vi "Initialize.vi"(7 "Serial Configuration":T1={"Baud Rate"=9600, "Parity"=0, "Data Bits"=8, "Stop Bits"=10, "Flow Control"=0} {"Flow Control" items=["None", "XON/XOFF", "RTS/CTS", "XON/XOFF & RTS/CTS", "DTR/DSR", "XON/XOFF & DTR/DSR"]; "Stop Bits" items=["1.0"=10, "1.5"=15, "2.0"=20]; "Data Bits" items=["7"=7, "8"=8]; "Parity" items=["None", "Odd", "Even", "Mark", "Space"]; "Baud Rate" items=["300"=300, "600"=600, "1200"=1200, "2400"=2400, "4800"=4800, "9600"=9600, "19200"=19200]}, 8 "error in (no error)":errorcluster, 9 "Reset (True)":bool=TRUE, 10 "ID Query (True)":bool=TRUE, 11 "VISA resource name":refnum<visa-resource-name>) -> (0 "error out":errorcluster, 3 "VISA resource name out":refnum<visa-resource-name>)   [LabVIEW 2014, in "Fluke 884X Series.lvlib"]
doc: "Establishes communication with the instrument and optionally performs an instrument identification query and/or an instrument reset. It also places the instrument in a default state needed for other instrument driver operations. Therefore, call this VI before calling other instrument driver VIs for this instrument. Generally, you need to call the <B>Initialize VI</B> only once at the beginning of an application."
uses:
  Fluke 884X Series.lvlib
panel:
  # "(c) 2007 National Instruments.  ALL RIGHTS RESERVED."
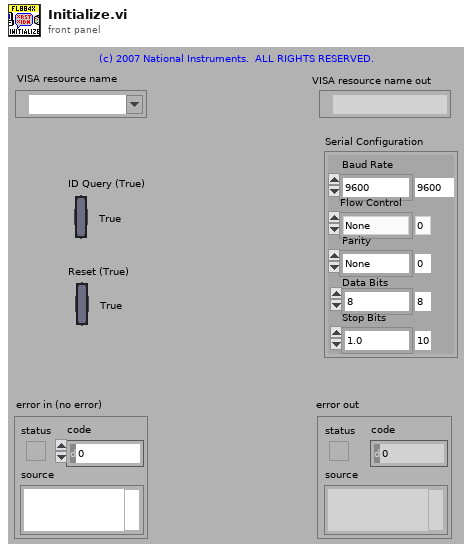
[diagram p1: front panel]
types:
  T1 = cluster{"Baud Rate":u32, "Parity":u16, "Data Bits":u16, "Stop Bits":u16, "Flow Control":u16}
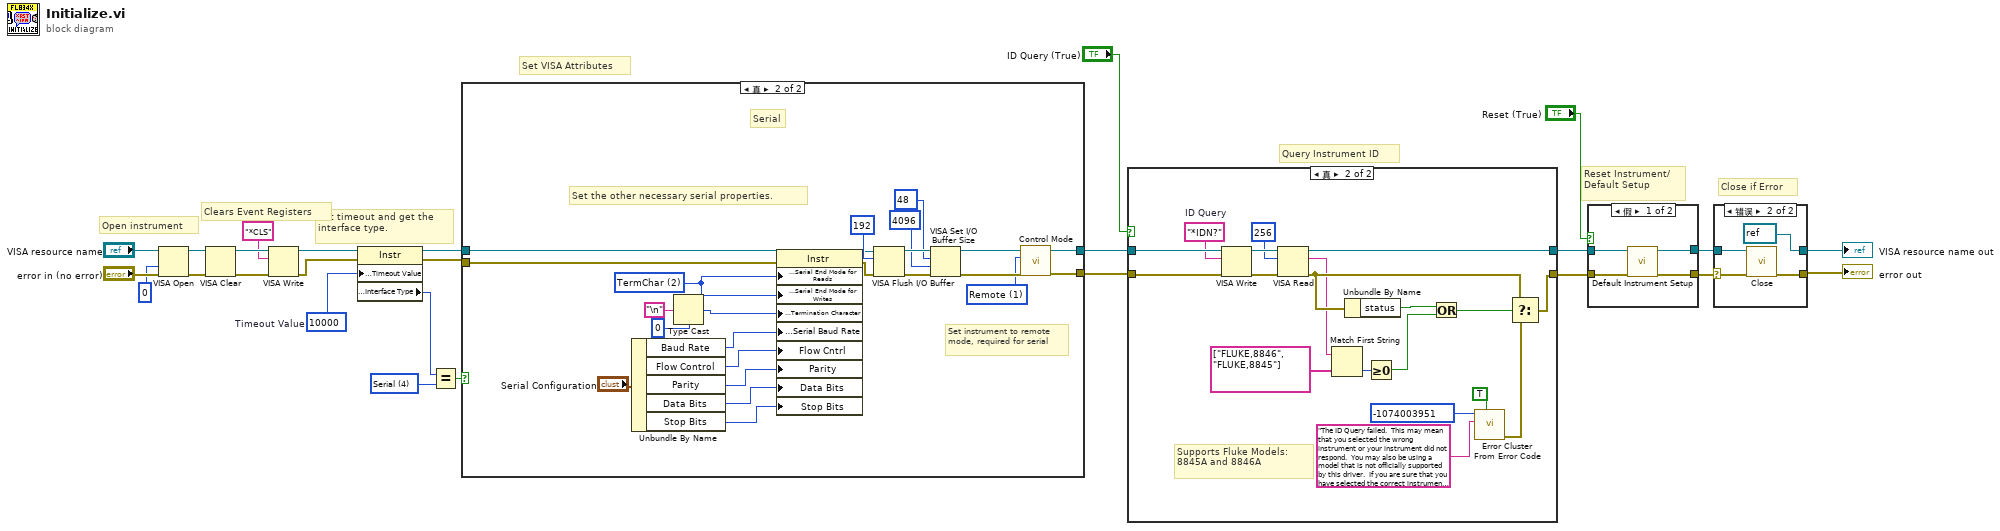
[diagram p0: block diagram]
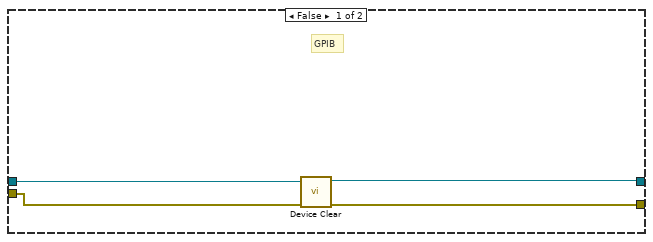
[diagram p3: hidden frame]
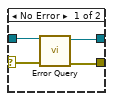
[diagram p4: hidden frame]
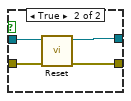
[diagram p5: hidden frame]
diagram:
  w20 = u16 4 items=["GPIB"=1, "VXI"=2, "GPIB-VXI"=3, "Serial"=4, "PXI"=5, "TCPIP"=6, "USB"=7] ("Interface Information:Interface Type")
  w22 = u32 10000  # Timeout Value
  # "Clears Event Registers"
  # "Set VISA Attributes"
  # "Set timeout and get the\ninterface type."
  # "Close if Error"
  # "Query Instrument ID"
  # "Reset Instrument/\nDefault Setup"
  # "Open instrument"
  n1 = VISA Open(access mode=u32 0, error in (no error)="error in (no error)", VISA resource name="VISA resource name") -> (VISA resource name=w8:refnum<visa-resource-name>, error out=w9:errorcluster)  [unwired: 2 in]
  n2 = VISA Clear(VISA resource name=w8, error in (no error)=w9) -> (VISA resource name out=w5:refnum<visa-resource-name>, error out=w4:errorcluster)
  n3 = VISA Write(VISA resource name=w5, write buffer="*CLS", error in (no error)=w4) -> (VISA resource name out=w2:refnum<visa-resource-name>, error out=w1:errorcluster)  [unwired: 1 out]
  n4 = property on="Property Node" class="Instr"(reference=w2, error in=w1, "General Settings:Timeout Value"=w22) -> (reference out=w11:refnum<visa-resource-name>, error out=w10:errorcluster, "Interface Information:Interface Type"=w23:u16)
  n5 = Equal?(x=w23, y=w20) -> (x = y?=w21:bool)
  n6 = case shown="真" w21 {
    tunnel: [w28 w33] -> w14
    tunnel: [w27 w32] -> w12
    tunnel: w11 -> [w30 w54]
    tunnel: w10 -> [w29 w53]
    frame False {
      # "GPIB"
      n7 = call "Device Clear.vi"("error in (no error)"=w29, "VISA Resource Name"=w30) -> ("error out"=w27:errorcluster, "VISA Resource Out"=w28:refnum<visa-resource-name>)  [unwired: 8 in]
    }
    frame True {
      w31 = u16 1 items=["Local", "Remote", "Remote with Lock"] ("Control Mode (0:Local)")
      w46 = u16 2 items=["None", "LastBit", "TermChar"] ("Serial Settings:Serial End Mode for Reads")
      # "Set instrument to remote mode, required for serial"
      # "Set the other necessary serial properties."
      # "Serial"
      n8 = Unbundle By Name("Serial Configuration") -> ("Baud Rate"=w40:u32, "Flow Control"=w39:u16, "Parity"=w38:u16, "Data Bits"=w37:u16, "Stop Bits"=w36:u16)
      n9 = Type Cast(type=u8 0, x="\n" ("Line Feed Constant")) -> (*(type *) &x=w47:u8)
      n10 = property on="Property Node" class="Instr"(reference=w54, error in=w53, "Serial Settings:Serial End Mode for Reads"=w46, "Serial Settings:Serial End Mode for Writes"=w46, "Message Based Settings:Termination Character"=w47, "Serial Settings:Serial Baud Rate"=w40, "Flow Cntrl"=w39, "Parity"=w38, "Data Bits"=w37, "Stop Bits"=w36) -> (reference out=w43:refnum<visa-resource-name>, error out=w42:errorcluster)
      n11 = VISA Flush I/O Buffer(VISA resource name=w43, mask (16)=u16 192, error in (no error)=w42) -> (VISA resource name out=w52:refnum<visa-resource-name>, error out=w51:errorcluster)
      n12 = VISA Set I/O Buffer Size(VISA resource name=w52, mask (16)=u16 48, size (4096)=u32 4096 ("size (0)"), error in (no error)=w51) -> (VISA resource name out=w35:refnum<visa-resource-name>, error out=w34:errorcluster)
      n13 = call "Control Mode.vi"("error in (no error)"=w34, "Control Mode (0:Local)"=w31, "VISA Resource Name"=w35) -> ("error out"=w32:errorcluster, "VISA Resource Out"=w33:refnum<visa-resource-name>)  [unwired: 7 in]
    }
  }
  n14 = case shown="真" "ID Query (True)" {
    tunnel: [w55 w75] -> w6
    tunnel: [w56 w72] -> w7
    tunnel: w14 -> [w56 w73]
    tunnel: w12 -> [w55 w74]
    frame False {
    }
    frame True {
      w68 = "*IDN?"  # ID Query
      # "Supports Fluke Models:\n8845A and 8846A"
      n15 = VISA Write(VISA resource name=w73, write buffer=w68, error in (no error)=w74) -> (VISA resource name out=w71:refnum<visa-resource-name>, error out=w70:errorcluster)  [unwired: 1 out]
      n16 = VISA Read(VISA resource name=w71, byte count=u32 256, error in (no error)=w70) -> (VISA resource name out=w72:refnum<visa-resource-name>, read buffer=w58:string, error out=w62:errorcluster)  [unwired: 1 out]
      n17 = Match First String(2:string[] ["FLUKE,8846", "FLUKE,8845"], 3:w58) -> (0:w63:i32)  [unwired: 1 out]
      n18 = Unbundle By Name(w62) -> ("status"=w61:bool)
      n19 = Greater Or Equal To 0?(x=w63) -> (x >= 0?=w60:bool)
      n20 = Or(x=w61, y=w60) -> (x .or. y?=w59:bool)
      n21 = call <vilib>:"Error Cluster From Error Code.vi"("show call chain? (False)"=TRUE, "error message (\"\")"="The ID Query failed.  This may mean that you selected the wrong instrument or your instrument did not respond.  You may also be using a model that is not officially supported by this driver.  If you are sure that you have selected the correct instrument and it is responding, try disabling the ID Query." ("Source (VI Name)"), "error code (0)"=-1074003951 ("Code")) -> ("error out"=w67:errorcluster)  [unwired: 6 in]
      n22 = Select(t=w62, s=w59, f=w67) -> (s? t:f=w75:errorcluster)
    }
  }
  n23 = case shown="假" "Reset (True)" {
    tunnel: w6 -> [w78 w80]
    tunnel: [w76 w83] -> w16
    tunnel: w7 -> [w79 w81]
    tunnel: [w77 w82] -> w17
    frame False {
      n24 = call "Default Instrument Setup.vi"("error in (no error)"=w78, "VISA resource name"=w79) -> ("error out"=w76:errorcluster, "VISA resource name out"=w77:refnum<visa-resource-name>)  [unwired: 8 in]
    }
    frame True {
      n25 = call "Reset.vi"("error in (no error)"=w80, "VISA resource name"=w81) -> ("error out"=w83:errorcluster, "VISA resource name out"=w82:refnum<visa-resource-name>)  [unwired: 8 in]
    }
  }
  n26 = case shown="错误" w16 {
    selector: w16 -> [w86 w89]
    tunnel: w17 -> [w87 w90]
    tunnel: [w85 refnum<visa-resource-name> refnum ("VISA resource name out")] -> w18
    tunnel: [w84 w91] -> w13
    frame No Error {
      n27 = call "Error Query.vi"("error in (no error)"=w86, "VISA resource name"=w87) -> ("error out"=w84:errorcluster, "VISA resource name out"=w85:refnum<visa-resource-name>)  [unwired: 6 in, 2 out]
    }
    frame Error {
      n28 = call "Close.vi"("error in (no error)"=w89, "VISA resource name"=w90) -> ("error out"=w91:errorcluster)  [unwired: 9 in]
    }
  }
  "VISA resource name out" <- w18
  "error out" <- w13
